vi "afslaan_proberen_deel2(SubVI).vi"(4 "stop 3":bool, 5 "stop":bool, 6 "stop 2":bool, 7 "universele stop":bool, 8 "OK Button":bool, 11 "element":string) -> ()   [LabVIEW 2019]
uses:
  <vilib>/myRIO/Express VI/Onboard IO/PWM/PWM Express VI.xnode
  <vilib>/myRIO/Instrument Drivers/Onboard IO/PWM/vis/Set Duty Cycle and Frequency.vi
  <vilib>/myRIO/Instrument Drivers/Onboard IO/PWM/PWM.lvlib
  <vilib>/myRIO/Instrument Drivers/Onboard IO/PWM/typedefs/PWM Configuration.ctl
  <vilib>/myRIO/Common/Instrument Driver Framework/myRIO v1.0/PWM/typedefs/PWM Channels Enum.ctl
  <vilib>/myRIO/Common/Instrument Driver Framework/Utilities/typedefs/Generic FPGA Reference.ctl
  <vilib>/myRIO/Common/Instrument Driver Framework/Utilities/typedefs/myRIO v1.0 Reference.ctl
  <vilib>/myRIO/Common/Instrument Driver Framework/Utilities/typedefs/Hardware Version Enum.ctl
  <vilib>/myRIO/Common/Instrument Driver Framework/Utilities/typedefs/myRIO Generic Hardware Reference.ctl
  <vilib>/myRIO/Instrument Drivers/Onboard IO/PWM/typedefs/PWM Reference.ctl
  <vilib>/myRIO/Instrument Drivers/Onboard IO/PWM/vis/myRIO PWM Open.xnode
  <vilib>/myRIO/Common/Instrument Driver Framework/Utilities/vis/Is FPGA Ref Available.vi
  <vilib>/myRIO/Common/Instrument Driver Framework/myRIO v1.0/PWM/vis/myRIO v1.1 Open PWM.vi
  <vilib>/userDefined/High Color/nirio_resource_hc.ctl
panel:
  out "rechtermotor:d":dbl=0.4
  out "linkermotor: d":dbl=0.4
  out "x*y 2":dbl
  out "x*y":dbl
  in  "error in (no error)":errorcluster
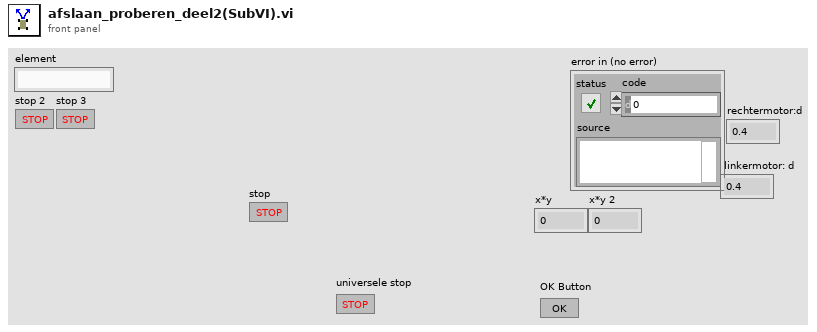
[diagram p1: front panel]
types:
  T1 = typedef "PWM.lvlib/PWM Reference.ctl" = cluster{"myRIO Reference":T2, "PWM Channels Enum":T6, "PWM Configuration":T7}
  T2 = typedef "myRIO Generic Hardware Reference.ctl" = cluster{"myRIO Model":T3, "myRIO Hardware Reference":T4}
  T3 = typedef "Hardware Version Enum.ctl" = enum16{"Unknown", "myRIO-1900", "myRIO-1950", "roboRIO", "NI ELVIS RIO CM", "ELVIS III"}
  T4 = typedef "myRIO v1.0 Reference.ctl" = cluster{"Generic FPGA Reference":T5, "Allow multiple opens":bool}
  T5 = typedef "Generic FPGA Reference.ctl" = refnum<k20>
  T6 = typedef "PWM Channels Enum.ctl" = enum16{"Not Connected", "C/PWM0", "C/PWM1", "A/PWM0", "A/PWM1", "A/PWM2", "A/PWM3", "A/PWM4", "A/PWM5", "A/PWM6", "A/PWM7", "A/PWM8", "A/PWM9", "A/PWM10", "A/PWM11", "A/PWM12", "A/PWM13", "A/PWM14", "A/PWM15", "A/PWM16", "A/PWM17", "A/PWM18", "A/PWM19", "B/PWM0", "B/PWM1", "B/PWM2", "B/PWM3", "B/PWM4", "B/PWM5", "B/PWM6", "B/PWM7", "B/PWM8", "B/PWM9", "B/PWM10", "B/PWM11", "B/PWM12", "B/PWM13", "B/PWM14", "B/PWM15", "B/PWM16", "B/PWM17", "B/PWM18", "B/PWM19", "PWM/PWM0", "PWM/PWM1", "PWM/PWM2", "PWM/PWM3", "PWM/PWM4", "PWM/PWM5", "PWM/PWM6", "PWM/PWM7", "PWM/PWM8", "PWM/PWM9"}
  T7 = typedef "PWM.lvlib/PWM Configuration.ctl" = cluster{"Frequency":dbl, "Duty Cycle":dbl}
  T8 = typedef "nirio_resource_hc.ctl" = tag
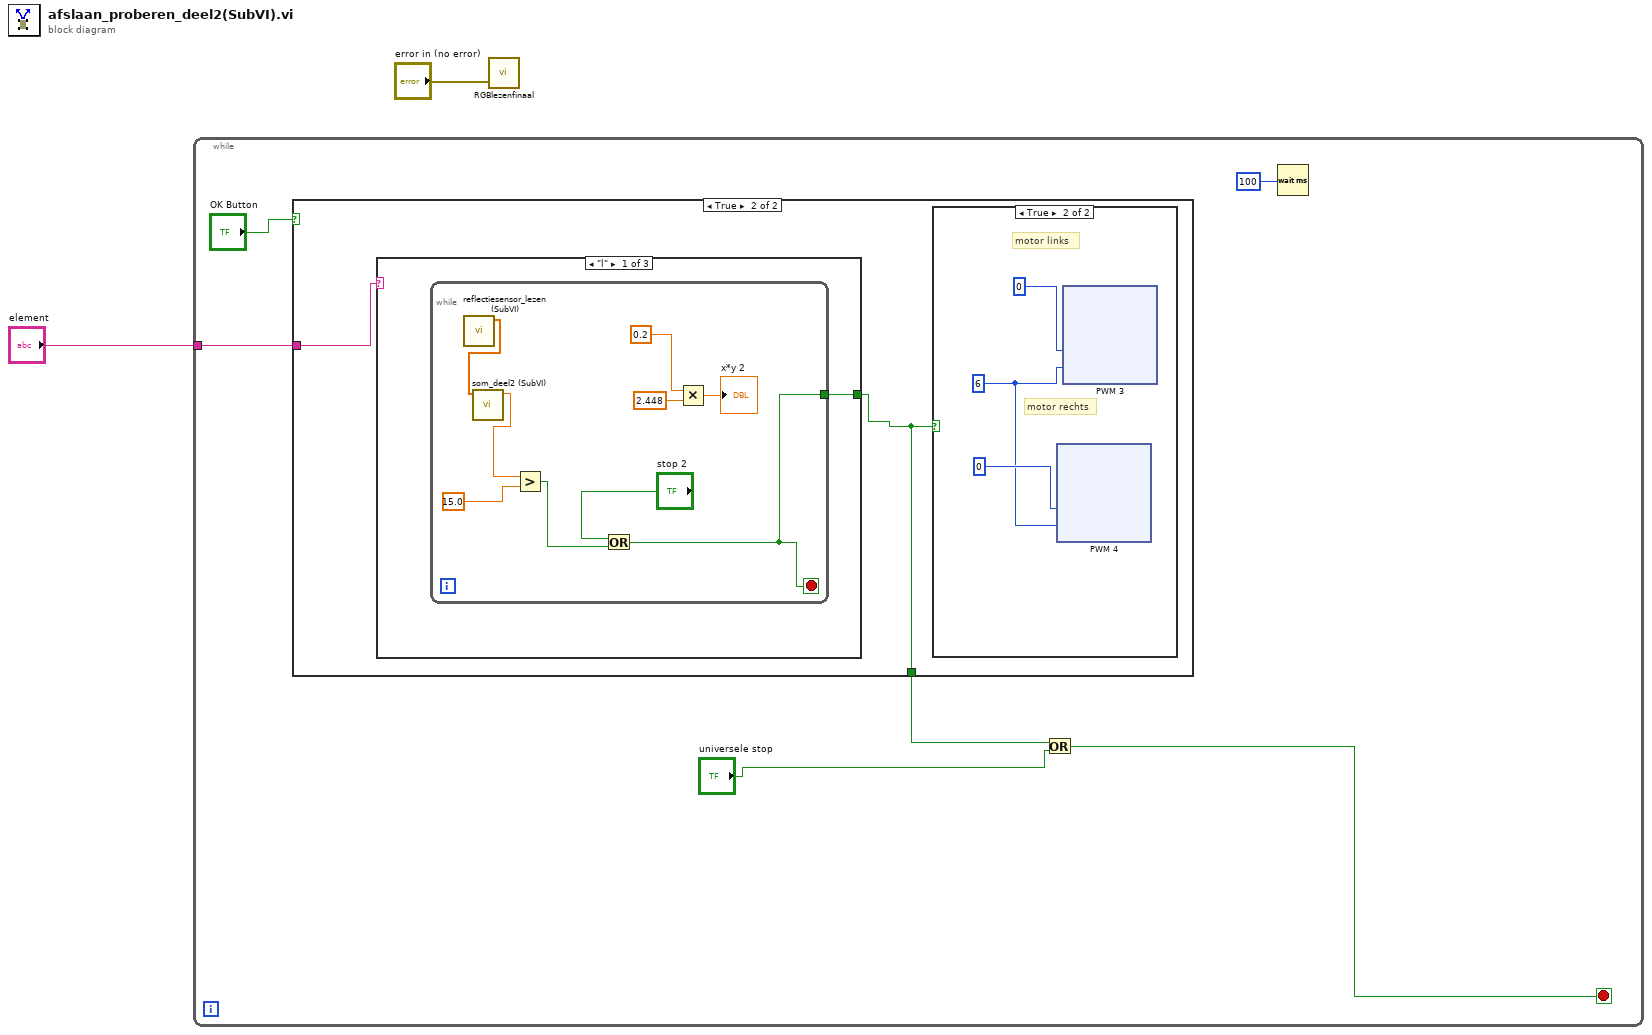
[diagram p0: block diagram]
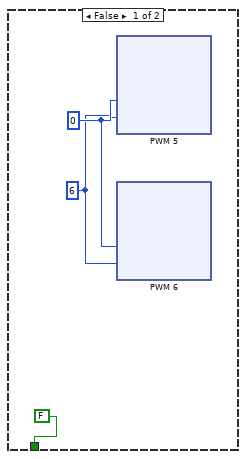
[diagram p2: hidden frame]
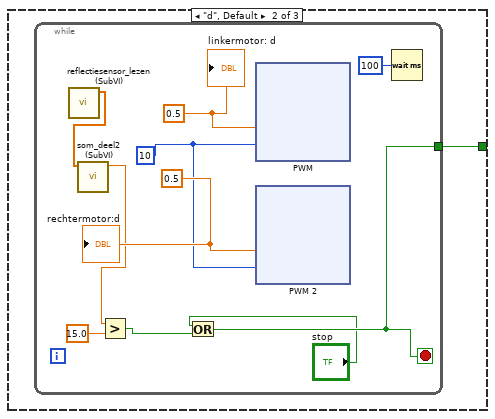
[diagram p3: hidden frame]
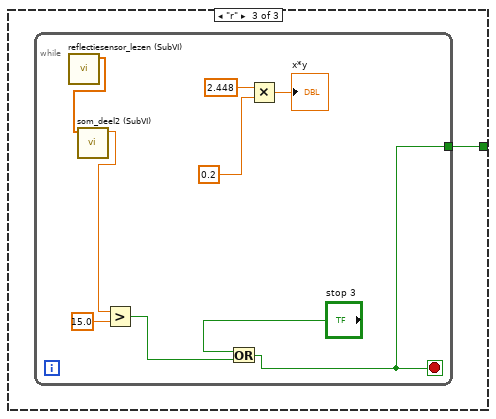
[diagram p4: hidden frame]
diagram:
  n1 = while {
    tunnel: "element" -> [w4]
    stop <- w6 stop-if-true
    n2 = case shown="True" "OK Button" {
      tunnel: [FALSE w83] -> w7
      tunnel: w4 -> [_ w82]
      frame False {
        w9 = 6
        w10 = 0
        n3 = xnode "PWM 5"("Duty Cycle"=w10, "Frequency [Hz]"=w9) -> ()  [unwired: 1 in, 1 out]
        n4 = xnode "PWM 6"("Duty Cycle"=w10, "Frequency [Hz]"=w9) -> ()  [unwired: 1 in, 1 out]
      }
      frame True {
        n5 = case shown="\"l\"" w82 {
          tunnel: [w84 w94 w175] -> w83
          frame "l" {
            n6 = while {
              tunnel: [w91] -> w84
              stop <- w91 stop-if-true
              n7 = call "reflectiesensor_lezen (SubVI).vi"() -> ("Values"=w88:dbl[])  [unwired: 11 in]
              n8 = call "som_deel2 (SubVI).vi"("array"=w88) -> ("x+y"=w86:dbl)  [unwired: 10 in]
              n9 = Greater?(x=w86, y=15.0) -> (0:w85:bool)
              n10 = Or(x="stop 2", y=w85) -> (x .or. y?=w91:bool)
              n11 = Multiply(x=0.2, y=2.448) -> (x*y=→"x*y 2":dbl)
            }
          }
          frame "d", Default {
            n12 = while {
              tunnel: [w104] -> w94
              stop <- w104 stop-if-true
              w101 = 10
              w102 = 0.5
              w103 = 0.5
              n13 = call "reflectiesensor_lezen (SubVI).vi"() -> ("Values"=w96:dbl[])  [unwired: 11 in]
              n14 = call "som_deel2 (SubVI).vi"("array"=w96) -> ("x+y"=w95:dbl)  [unwired: 10 in]
              n15 = Greater?(x=w95, y=15.0) -> (0:w97:bool)
              n16 = Or(x="stop", y=w97) -> (x .or. y?=w104:bool)
              n17 = xnode "PWM"("Duty Cycle"=w103, "Frequency [Hz]"=w101) -> ()  [unwired: 1 in, 1 out]
              n18 = xnode "PWM 2"("Duty Cycle"=w102, "Frequency [Hz]"=w101) -> ()  [unwired: 1 in, 1 out]
              n19 = Wait (ms)(milliseconds to wait=u32 100) -> ()  [unwired: 1 out]
              "linkermotor: d" <- w103
              "rechtermotor:d" <- w102
            }
          }
          frame "r" {
            n20 = while {
              tunnel: [w182] -> w175
              stop <- w182 stop-if-true
              n21 = call "reflectiesensor_lezen (SubVI).vi"() -> ("Values"=w179:dbl[])  [unwired: 11 in]
              n22 = call "som_deel2 (SubVI).vi"("array"=w179) -> ("x+y"=w177:dbl)  [unwired: 10 in]
              n23 = Greater?(x=w177, y=15.0) -> (0:w176:bool)
              n24 = Or(x="stop 3", y=w176) -> (x .or. y?=w182:bool)
              n25 = Multiply(x=2.448, y=0.2) -> (x*y=→"x*y":dbl)
            }
          }
        }
        n26 = case shown="True" w83 {
          frame False {
          }
          frame True {
            w185 = 6
            # "motor rechts"
            # "motor links"
            n27 = xnode "PWM 4"("Duty Cycle"=0, "Frequency [Hz]"=w185) -> ()  [unwired: 1 in, 1 out]
            n28 = xnode "PWM 3"("Duty Cycle"=0, "Frequency [Hz]"=w185) -> ()  [unwired: 1 in, 1 out]
          }
        }
      }
    }
    n29 = Or(x=w7, y="universele stop") -> (x .or. y?=w6:bool)
    n30 = Wait (ms)(milliseconds to wait=100) -> ()  [unwired: 1 out]
  }
  n31 = call "RGBlezenfinaal.vi"("error in (no error)"="error in (no error)") -> ()  [unwired: 2 in, 1 out]
